vi "PI_E709.vi"() -> ()   [LabVIEW 2012]
panel:
  in  "Exit":bool
  in  "Step number":dbl min=0.0 max=10000.0 step=100.0
  in  "Step size":dbl min=0.0 max=1.0 step=0.001
  out "Scan":bool
  out "Stop":bool
  in  "Cancel":bool
  in  "Scan":bool
  out "Stage names":string[](array[string])
  out "Position":dbl
  in  "Target":dbl min=0.0 max=100.0 step=0.1
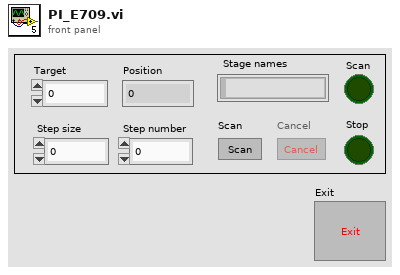
[diagram p1: front panel]
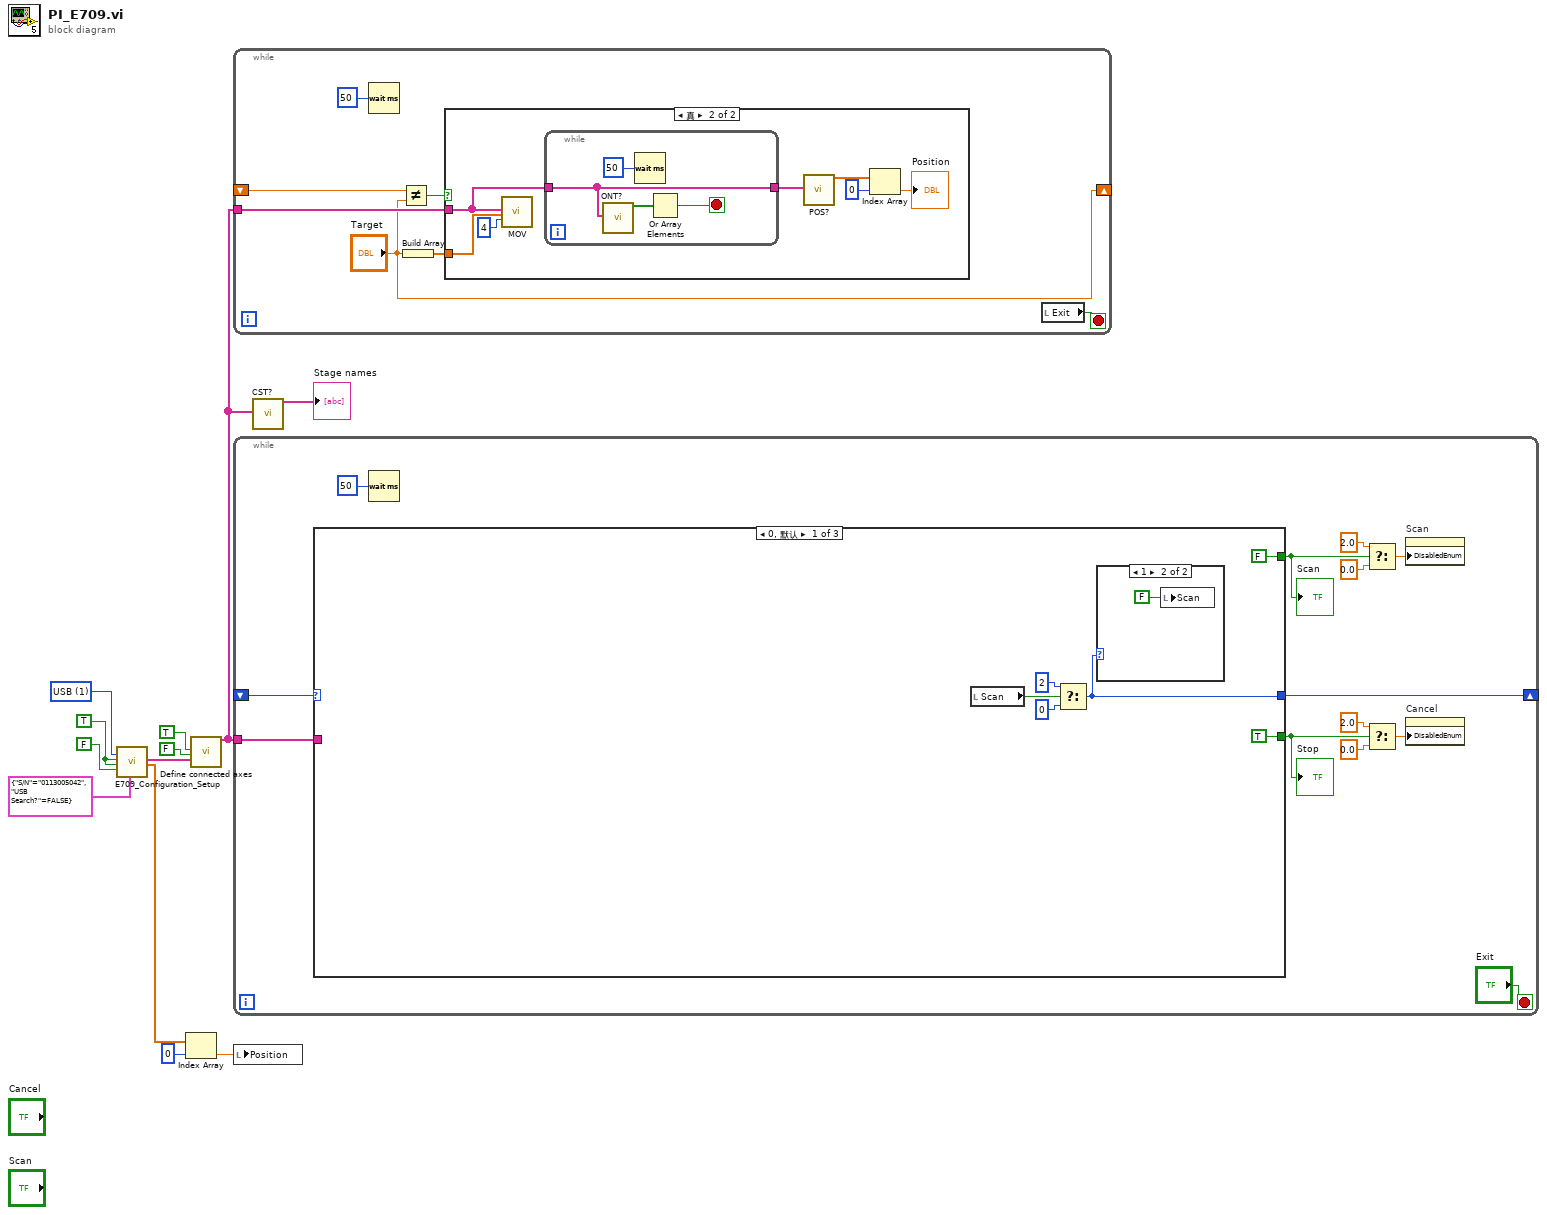
[diagram p0: block diagram]
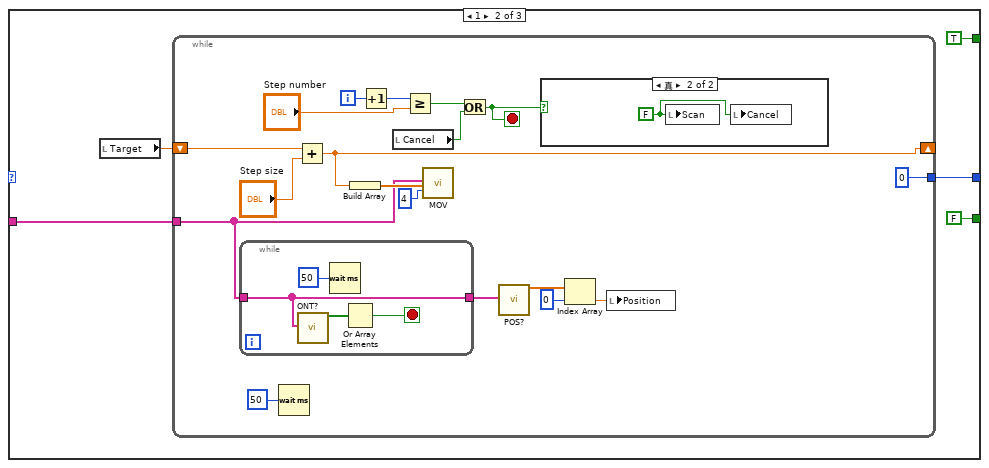
[diagram p3: hidden frame]
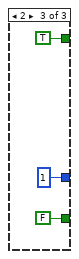
[diagram p5: hidden frame]
diagram:
  w1 = TRUE ("Connected?")
  w12 = u16 1 items=["RS232", "USB"] ("Interface")
  n1 = call "E709_Configuration_Setup.vi"("Interface"=w12, "Connected?"=w1, "Change servo status to ON?"=w1, "Perform autozero?"=FALSE, "USB settings"=cluster{"S/N":string, "USB Search?":bool} {"S/N"="0113005042", "USB Search?"=FALSE}) -> ("Conn. \nAxis"=w10:string[], "Position"=w6:dbl[])  [unwired: 9 in, 4 out]
  n2 = Index Array(array=w6, index=0 ("索引")) -> (element=w4:dbl)
  n3 = call "Define connected axes.vi"("Read from\ncontroller?"=TRUE ("Read from\ncontroller?"), "Invert\norder?"=FALSE ("Invert\norder?"), "Conn. axes"=w10) -> ("Conn. Axes out"=w2:string[])  [unwired: 15 in, 1 out]
  n4 = while {
    tunnel: w2 -> [w19]
    shift-right: ["Target"] -> _
    shift-left: _ -> [w18]
    stop <- w13 stop-if-true
    n5 = Wait (ms)(milliseconds to wait=u32 50 ("等待时间（毫秒）")) -> ()  [unwired: 1 out]
    n6 = Not Equal?(x=w18, y="Target") -> (x != y?=w17:bool)
    n7 = Build Array("Target") -> (w15:dbl[])
    n8 = case shown="真" w17 {
      tunnel: w19 -> [_ w25]
      tunnel: w15 -> [_ w24]
      frame False {
      }
      frame True {
        n9 = call "MOV.vi"("Axes to move"=w25, "Position values"=w24, "No.of digits"=i16 4) -> ()  [unwired: 16 in, 1 out]
        n10 = while {
          tunnel: w25 -> [w30]
          tunnel: [w30] -> w26
          stop <- w28 stop-if-true
          n11 = call "ONT?.vi"("Axes to query"=w30) -> ("Axis on target?"=w29:bool[])  [unwired: 17 in, 1 out]
          n12 = Wait (ms)(milliseconds to wait=u32 50 ("等待时间（毫秒）")) -> ()  [unwired: 1 out]
          n13 = Or Array Elements(Boolean array=w29) -> (logical OR=w28:bool)
        }
        n14 = call "POS?.vi"("Axes to query"=w26) -> ("Position"=w22:dbl[])  [unwired: 17 in, 1 out]
        n15 = Index Array(array=w22, index=0 ("索引")) -> (element=→"Position":dbl)
      }
    }
    n16 = local read "Exit"() -> (w13:bool)
  }
  n17 = while {
    shift-right: [w41] -> _
    shift-left: _ -> [w42]
    tunnel: w2 -> [w31]
    stop <- "Exit" stop-if-true
    n18 = case shown="0, 默认" w42 {
      tunnel: [w44 w54 1] -> w41
      tunnel: [TRUE ("Scan") FALSE FALSE] -> w39
      tunnel: [FALSE ("Scan") TRUE TRUE] -> w40
      tunnel: w31 -> [_ w51 _]
      frame 0, Default {
        n19 = local read "Scan"() -> (w49:bool)
        n20 = Select(t=2, s=w49, f=0) -> (s? t:f=w44:i32)
        n21 = case shown="1" w44 {
          frame 0, Default {
          }
          frame 1 {
            n22 = local write "Scan"(FALSE ("Scan")) -> ()
          }
        }
      }
      frame 1 {
        n23 = local read "Target"() -> (w55:dbl)
        n24 = while {
          shift-right: [w62] -> _
          shift-left: w55 -> [w70]
          tunnel: [0] -> w54
          tunnel: w51 -> [w57]
          i -> [w65]
          stop <- w68 stop-if-true
          n25 = while {
            tunnel: [w74] -> w58
            tunnel: w57 -> [w74]
            stop <- w75 stop-if-true
            n26 = call "ONT?.vi"("Axes to query"=w74) -> ("Axis on target?"=w77:bool[])  [unwired: 17 in, 1 out]
            n27 = Wait (ms)(milliseconds to wait=u32 50 ("等待时间（毫秒）")) -> ()  [unwired: 1 out]
            n28 = Or Array Elements(Boolean array=w77) -> (logical OR=w75:bool)
          }
          n29 = Wait (ms)(milliseconds to wait=u32 50 ("等待时间（毫秒）")) -> ()  [unwired: 1 out]
          n30 = Add(x=w70, y="Step size") -> (x+y=w62:dbl)
          n31 = Build Array(w62) -> (w61:dbl[])
          n32 = Increment(x=w65) -> (x+1=w64:i32)
          n33 = local read "Cancel"() -> (w73:bool)
          n34 = Greater Or Equal?(x=w64, y="Step number") -> (x >= y?=w72:bool)
          n35 = call "MOV.vi"("Axes to move"=w57, "Position values"=w61, "No.of digits"=i16 4) -> ()  [unwired: 16 in, 1 out]
          n36 = Or(x=w72, y=w73) -> (x .or. y?=w68:bool)
          n37 = call "POS?.vi"("Axes to query"=w58) -> ("Position"=w60:dbl[])  [unwired: 17 in, 1 out]
          n38 = case shown="真" w68 {
            frame False {
            }
            frame True {
              w78 = FALSE
              n39 = local write "Scan"(w78) -> ()
              n40 = local write "Cancel"(w78) -> ()
            }
          }
          n41 = Index Array(array=w60, index=0 ("索引")) -> (element=w56:dbl)
          n42 = local write "Position"(w56) -> ()
        }
      }
      frame 2 {
      }
    }
    "Scan" <- w40
    "Stop" <- w39
    n43 = Wait (ms)(milliseconds to wait=u32 50 ("等待时间（毫秒）")) -> ()  [unwired: 1 out]
    n44 = Select(t=2.0, s=w40, f=0.0) -> (s? t:f=w33:dbl)
    n45 = Select(t=2.0, s=w39, f=0.0) -> (s? t:f=w32:dbl)
    n46 = property on="Scan" class="Bool (严格)"("DisabledEnum"=w33) -> ()  [unwired: 2 in, 2 out]
    n47 = property on="Cancel" class="Bool (严格)"("DisabledEnum"=w32) -> ()  [unwired: 2 in, 2 out]
  }
  n48 = local write "Position"(w4) -> ()
  n49 = call "CST?.vi"("Axes to query"=w2) -> ("Stage names"=→"Stage names":string[])  [unwired: 17 in, 1 out]
